vi "Launcher.vi"   [LabVIEW 2024, in "Application.lvlib"]
uses:
  Application.lvlib
  Main.vi
  Modules/Data Base/DataBase - Top VI.vi
  Modules/Error Handler/Error - Top VI.vi
  Modules/Session Scanner/Scanner - Top VI.vi
  Modules/User Interface/UI - Top VI.vi
  Modules/Data Base/Data Base.lvlib
  Modules/Error Handler/Error Handler.lvlib
  Modules/Session Scanner/Session Scanner.lvlib
  Modules/User Interface/User Interface.lvlib
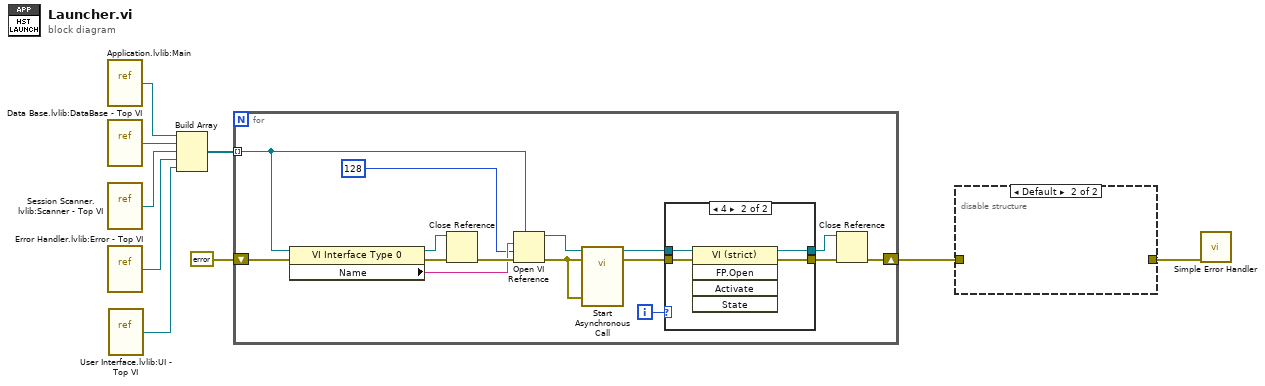
[diagram p0: block diagram]
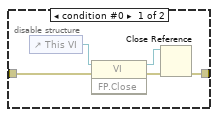
[diagram p3: hidden frame]
diagram:
  n1 = vi-ref "Application.lvlib:Main.vi"() -> (w5:refnum<vi>)
  n2 = vi-ref "Data Base.lvlib:DataBase - Top VI.vi"() -> (w4:refnum<vi>)
  n3 = vi-ref "Session Scanner.lvlib:Scanner - Top VI.vi"() -> (w3:refnum<vi>)
  n4 = vi-ref "Error Handler.lvlib:Error - Top VI.vi"() -> (w2:refnum<vi>)
  n5 = vi-ref "User Interface.lvlib:UI - Top VI.vi"() -> (w1:refnum<vi>)
  n6 = Build Array(w5, w4, w3, w2, w1) -> (w6:refnum<vi>[])
  n7 = for {
    shift-right: [w12] -> w8
    shift-left: errorcluster {"status"=FALSE, "code"=0, "source"=""} ("error out") -> [w19]
    tunnel: w6 -> [w18] mode=indexing
    i -> [w21]
    n8 = property class="VI Interface Type 0"(reference=w18, error in=w19) -> (reference out=w16:refnum<vi>, error out=w17:errorcluster, "Name"=w14:string)
    n9 = Close Reference(reference=w16, error in (no error)=w17) -> (error out=w15:errorcluster)
    n10 = Open VI Reference(type specifier VI Refnum (for type only)=w18, vi path=w14, options=128, error in (no error)=w15) -> (vi reference=w20:refnum<vi>, error out=w24:errorcluster)  [unwired: 2 in]
    n11 = call-by-ref "Start Asynchronous Call"(reference=w20, error in=w24, "error in"=w24) -> (reference out=w13:refnum<vi>, error out=w23:errorcluster)  [unwired: 10 in, 1 out]
    n12 = case shown="4" w21 {
      tunnel: w13 -> [w25 w30]
      tunnel: w23 -> [w26 w29]
      tunnel: [w26 w28] -> w22
      tunnel: [w25 w27] -> w11
      frame Default {
      }
      frame 4 {
        n13 = invoke class="VI (strict)" method="FP.Open"(reference=w30, error in=w29) -> (reference out=w27:refnum<vi>, error out=w28:errorcluster)  [unwired: 3 in, 3 out]
      }
    }
    n14 = Close Reference(reference=w11, error in (no error)=w22) -> (error out=w12:errorcluster)
  }
  n15 = disable-structure shown="Default" {
    disable-tunnel: w8 -> [w35 _]
    disable-tunnel: [w32 _] -> w7
    frame condition #0 {
      n16 = control-ref of="This VI"() -> (w33:refnum<vi>)
      n17 = invoke class="VI" method="FP.Close"(reference=w33, error in=w35) -> (reference out=w31:refnum<vi>, error out=w34:errorcluster)  [unwired: 1 in, 1 out]
      n18 = Close Reference(reference=w31, error in (no error)=w34) -> (error out=w32:errorcluster)
    }
    frame condition #1 (active) {
    }
  }
  n19 = call <vilib>:"Simple Error Handler.vi"("error in (no error)"=w7) -> ()  [unwired: 4 in, 5 out]
